vi "Init Response.vi"(8 "error in (no error)":errorcluster, 10 "Result":refnum<class "Acquired Result.lvclass">, 11 "Measure Controller in":refnum<class "Process Controller.lvclass">) -> (0 "error out":errorcluster, 3 "Measure Controller out":refnum<class "Process Controller.lvclass">)   [LabVIEW 2016, in "Process Controller.lvclass"]
uses:
  Process Controller.lvclass
  NHMFL_Core/Libraries/Instruments/Results/Acquired Result/Acquired Result.lvclass
  C:/github/LabActor/Worker/Worker.lvclass
  C:/github/LabActor/Template Module/Template Module.lvclass
  Process Controller.lvclass/Process Controller.ctl
  NHMFL_Core/Libraries/Instruments/Instrument Driver/Worker State.ctl
  Worker/Worker.lvclass/Worker.ctl
  Template Module/Template Module.lvclass/Template Module.ctl
  Template Module/Write State.vi
  Template Module/Read Reply to.vi
  Worker/Read Cycle count.vi
  Read Repeat times.vi
  Template Module Messages/Result Reply Msg/Result Reply Msg.lvclass
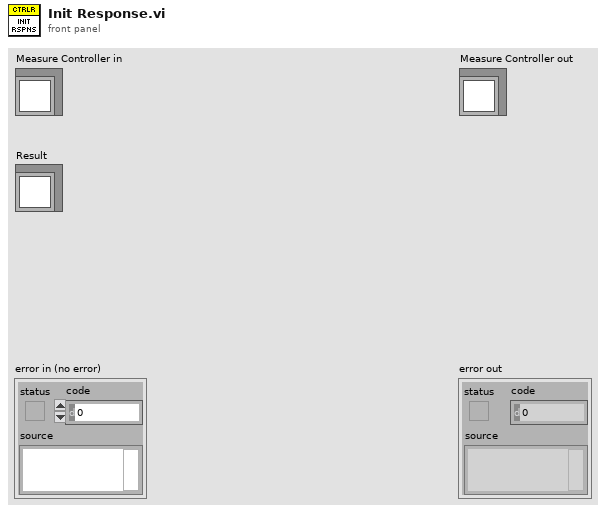
[diagram p1: front panel]
types:
  T1 = typedef "Worker State.ctl" = enum16{"Idle", "Starting", "Working", "Stopping"}
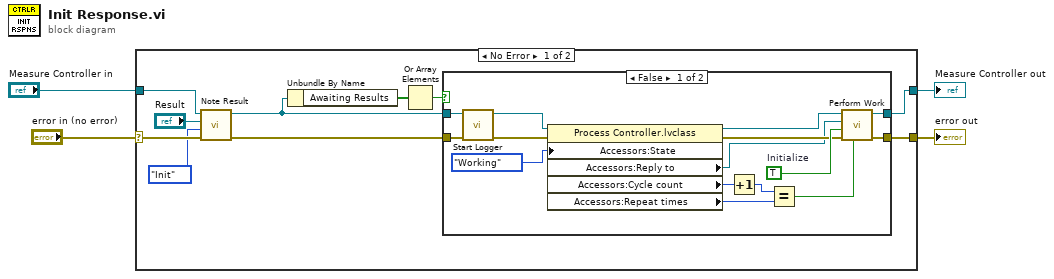
[diagram p0: block diagram]
diagram:
  n1 = case shown="No Error" "error in (no error)" {
    selector: "error in (no error)" -> [w13 w33]
    tunnel: [w6 w33] -> w3
    tunnel: [w8 w32] -> w1
    tunnel: "Measure Controller in" -> [w12 w32]
    frame No Error {
      n2 = call-dynamic "Note Result.vi"("error in (no error)"=w13, "Stage"=enum16{"Init", "Work"}."Init", "Acquired Result.lvclass"="Result", "Measure Controller in"=w12) -> ("error out"=w7:errorcluster, "Measure Controller out"=w9:refnum<class "Process Controller.lvclass">)  [unwired: 6 in]
      n3 = Unbundle By Name(w9) -> ("Awaiting Results"=w11:bool[])
      n4 = Or Array Elements(Boolean array=w11) -> (logical OR=w10:bool)
      n5 = case shown="False" w10 {
        tunnel: w9 -> [w27 w31]
        tunnel: [w29 w31] -> w8
        tunnel: w7 -> [w26 w30]
        tunnel: [w28 w30] -> w6
        frame False {
          w25 = TRUE  # Initialize
          n6 = call-dynamic "Start Logger.vi"("error in (no error)"=w26, "Measure Controller in"=w27) -> ("error out"=w22:errorcluster, "Measure Controller out"=w24:refnum<class "Process Controller.lvclass">)  [unwired: 6 in, 2 out]
          n7 = property class="Process Controller.lvclass"(reference=w24, error in=w22, "Accessors:State"=Worker_State."Working" ("State")) -> (reference out=w23:refnum<class "Process Controller.lvclass">, error out=w21:errorcluster, "Accessors:Reply to"=w16:refnum<class "Result Reply Msg.lvclass">, "Accessors:Cycle count"=w17:i32, "Accessors:Repeat times"=w20:i32)
          n8 = Increment(x=w17) -> (x+1=w19:i32)
          n9 = Equal?(x=w19, y=w20) -> (x = y?=w18:bool)
          n10 = call-dynamic "Perform Work.vi"("Last request"=w18, "error in (no error)"=w21, "Initialize"=w25, "Reply to"=w16, "Measure Controller in"=w23) -> ("error out"=w28:errorcluster, "Measure Controller out"=w29:refnum<class "Process Controller.lvclass">)  [unwired: 5 in]
        }
        frame True {
        }
      }
    }
    frame Error {
    }
  }
  "error out" <- w3
  "Measure Controller out" <- w1
